vi "Ins2182ARead_ver1.0.vi"(0 "VISA session":refnum<visa-resource-name>, 1 "error out":errorcluster) -> (2 "VISA session 2":refnum<visa-resource-name>, 3 "Numeric":dbl, 4 "error out 2":errorcluster)   [LabVIEW 2012]
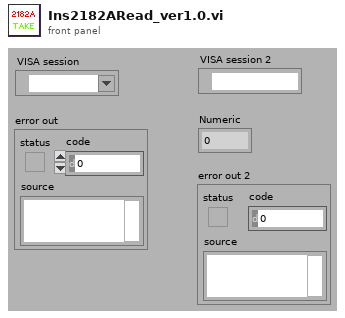
[diagram p1: front panel]
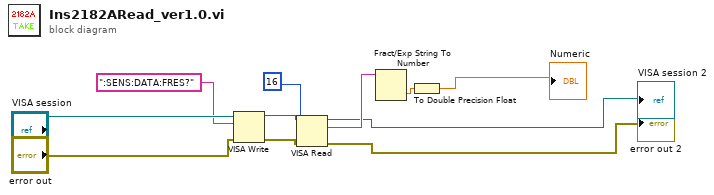
[diagram p0: block diagram]
diagram:
  n1 = VISA Write(VISA resource name="VISA session", write buffer=":SENS:DATA:FRES?", error in (no error)="error out") -> (VISA resource name out=w8:refnum<visa-resource-name>, error out=w9:errorcluster)  [unwired: 1 out]
  n2 = VISA Read(VISA resource name=w8, byte count=u32 16, error in (no error)=w9) -> (VISA resource name out=→"VISA session 2":refnum<visa-resource-name>, read buffer=w11:string, error out=→"error out 2":errorcluster)  [unwired: 1 out]
  n3 = Fract/Exp String To Number(string=w11) -> (number=w10:dbl)  [unwired: 3 in, 1 out]
  n4 = To Double Precision Float(number=w10) -> (double precision float=→"Numeric":dbl)
